vi "Test_Resolve Service.vi"() -> ()   [LabVIEW 2020]
uses:
  Discovery_client/RPC Messages/NIMeasurementServices_ResolveServiceRequest.ctl
  Discovery_client/RPC Messages/NIMeasurementServices_ServiceLocation.ctl
  Discovery_client/Discovery_client.lvlib
panel:
  out "Response Data":T1
  in  "Request Data":T2
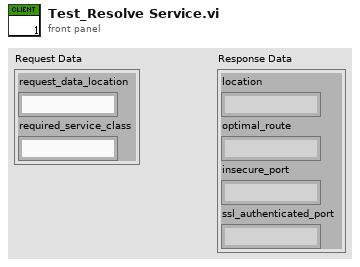
[diagram p1: front panel]
types:
  T1 = typedef "Discovery_client.lvlib/NIMeasurementServices_ServiceLocation.ctl" = cluster{"location":string, "optimal_route":string, "insecure_port":string, "ssl_authenticated_port":string}
  T2 = typedef "Discovery_client.lvlib/NIMeasurementServices_ResolveServiceRequest.ctl" = cluster{"request_data_location":string, "required_service_class":string}
  T3 = typedef "gprc-lvsupport-release.lvlib/grpcId.ctl" = u64
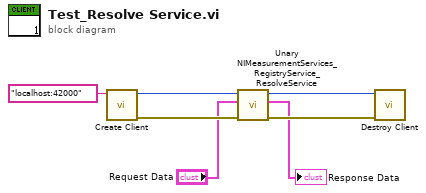
[diagram p0: block diagram]
diagram:
  n1 = call "Create Client.vi"("address"="localhost:42000") -> ("error out"=w5:errorcluster, "gRPC ID Out"=w6:T3)  [unwired: 9 in]
  n2 = call "Unary NIMeasurementServices_RegistryService_ResolveService.vi"("error in"=w5, "Request Data"="Request Data", "gRPC ID"=w6) -> ("error out"=w4:errorcluster, "Response Data"=→"Response Data":T1, "gRPC ID out"=w3:T3)  [unwired: 6 in]
  n3 = call "Destroy Client.vi"("error in"=w4, "gRPC ID"=w3) -> ()  [unwired: 9 in, 1 out]
